vi "simple stepper simulation.vi"() -> ()   [LabVIEW 2009]
panel:
  in  "Forward? (TRUE)":bool=TRUE
  out "current position":i32
  in  "milliseconds to wait":u32=100
  in  "stop":bool
  out "Coil charge":bool[](array[boolean])
  # "ON is positive\nOFF is negative"
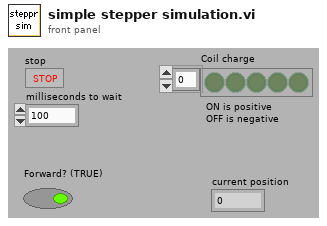
[diagram p1: front panel]
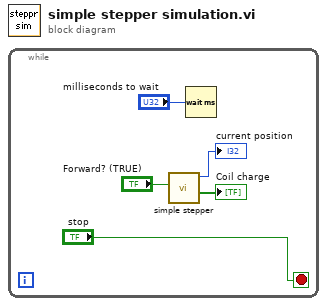
[diagram p0: block diagram]
diagram:
  n1 = while {
    stop <- "stop" stop-if-true
    n2 = call "simple stepper.vi"("Forward? (TRUE)"="Forward? (TRUE)") -> ("Coil charge"=→"Coil charge":bool[], "position"=→"current position":i32)  [unwired: 8 in, 1 out]
    n3 = Wait (ms)(milliseconds to wait="milliseconds to wait") -> ()  [unwired: 1 out]
  }
